vi "NewTaskItem.vi"(11 "TaskConfig":refnum<data-value>) -> ()   [LabVIEW 2025, in "DAQ_Module.lvlib" / "DAQ_Module.lvclass"]
uses:
  DAQ_Module.lvclass
  DAQ_Config.ctl
  DAQ_Task_Config.ctl
  DAQ_HW_Type.ctl
  DAQ_Task_Type.ctl
  DAQ_SampleRateConfig.ctl
  DAQ_Module.lvclass/DAQ_Module.ctl
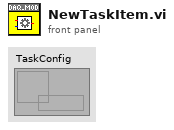
[diagram p1: front panel]
types:
  T1 = typedef "DAQ_Module.lvlib/DAQ_Module.lvclass/DAQ_Task_Config.ctl" = cluster{"Drive":T2, "TaskType":T3, "PhysicalChannels":string, "SampleRateConfiguration":T4, "ChannelConfig":map{string, cluster{"Name":string, "Config":string}}, "Enable":bool, "ShowPanel":bool}
  T2 = typedef "DAQ_Module.lvlib/DAQ_Module.lvclass/DAQ_HW_Type.ctl" = enum16{"NI_DAQmx", "Simulated_DAQ"}
  T3 = typedef "DAQ_Module.lvlib/DAQ_Module.lvclass/DAQ_Task_Type.ctl" = enum16{"AI", "Linear", "Angular", "AO"}
  T4 = typedef "DAQ_Module.lvlib/DAQ_Module.lvclass/DAQ_SampleRateConfig.ctl" = cluster{"SampleRate":dbl, "SamplesPerChannel":u32, "SamplesPerRead":i32, "SampleMode":i32, "Clock Source":string}
  T5 = typedef "DAQ_Module.lvlib/DAQ_Module.lvclass/DAQ_Config.ctl" = map{string, T1}
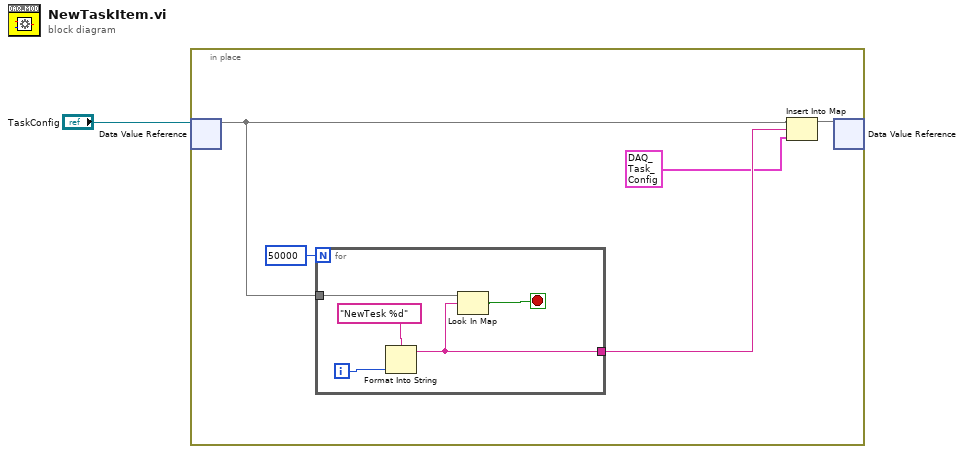
[diagram p0: block diagram]
diagram:
  n1 = in-place {
    n2 = in-place-dvr #1("TaskConfig") -> (w5:T5)  [unwired: 1 out]
    n3 = for {
      N: 50000 -> [_]
      tunnel: w5 -> [w11]
      tunnel: [w7] -> w4
      i -> [w8]
      stop <- w10 stop-if-true
      n4 = Format Into String(format string="NewTesk %d", w8) -> (resulting string=w7:string)  [unwired: 2 in, 1 out]
      n5 = Look In Map(map=w11, key=w7) -> (key not found?=w10:bool)  [unwired: 1 in, 1 out]
    }
    n6 = Insert Into Map(map in=w5, key=w4, value=T1 {"Drive"=enum."NI_DAQmx", "TaskType"=enum."AI", "PhysicalChannels"="/Dev1/ai0:3", "SampleRateConfiguration"={"SampleRate"=1000.0, "SamplesPerChannel"=1000, "SamplesPerRead"=200, "SampleMode"=10123, "Clock Source"="OnboardClock"}, "ChannelConfig"={}, "Enable"=TRUE, "ShowPanel"=FALSE} ("TaskConfig 2")) -> (map out=w2:T5)  [unwired: 2 out]
    n7 = in-place-dvr #1(w2) -> ()  [unwired: 2 out]
  }
